vi "HUI.vi"() -> ()   [LabVIEW 2016]
uses:
  <vilib>/measure/NI_MABase.lvlib
panel:
  out "Point processed":u32
  in  "Quant":i32=100
  in  "stop":bool
  out "DAC FREQ/CH, Hz":dbl
  out "String":string
  in  "STOP_RUN":bool
  in  "FREQ":dbl(knob)=100.0 scale=0.0..100000.0
  in  "SIZE":dbl(knob)=1.0 scale=0.0..5.0
  # "CHANNEL A"
  # "CHANNEL B"
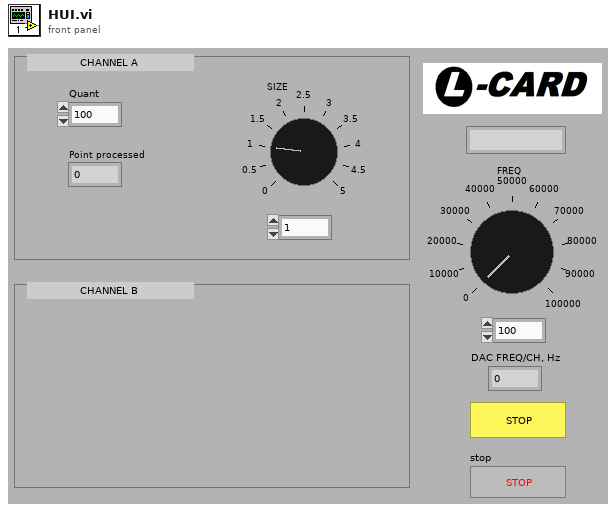
[diagram p1: front panel]
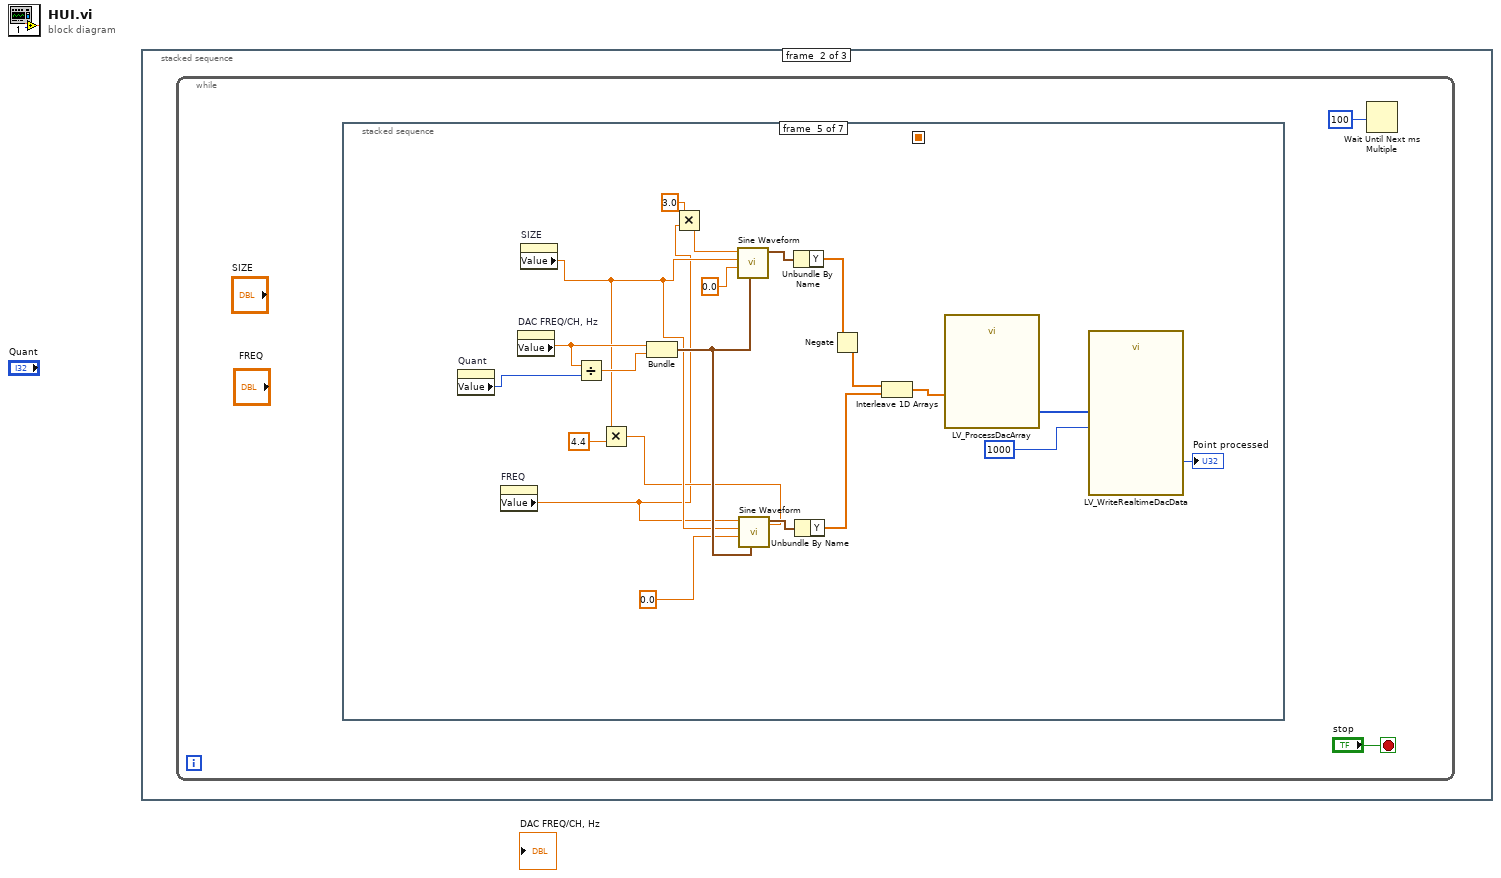
[diagram p0: block diagram]
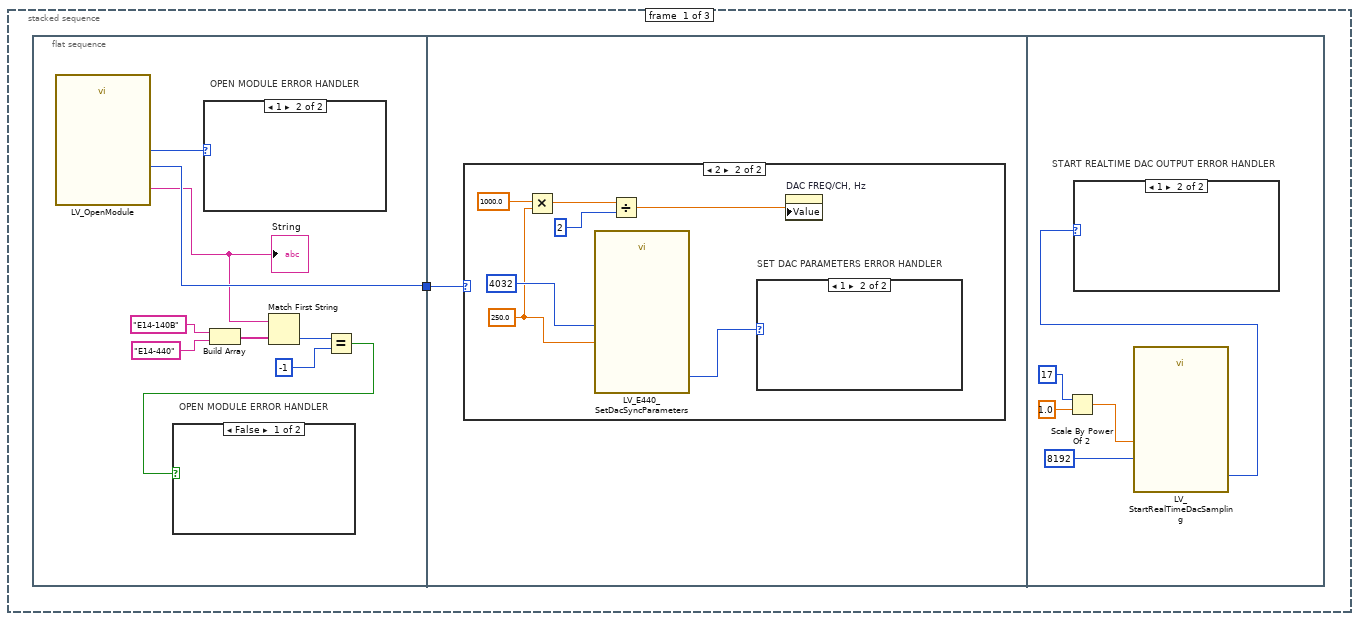
[diagram p2: hidden frame]
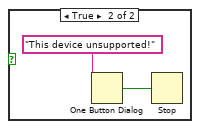
[diagram p3: hidden frame]
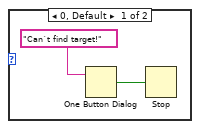
[diagram p4: hidden frame]
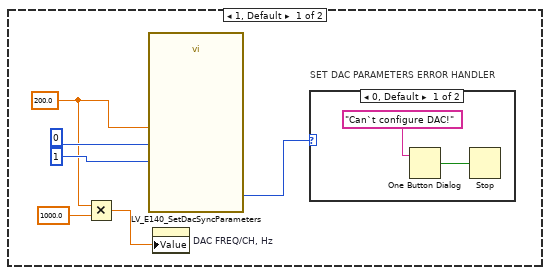
[diagram p5: hidden frame]
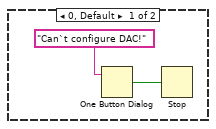
[diagram p7: hidden frame]
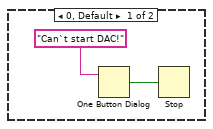
[diagram p8: hidden frame]
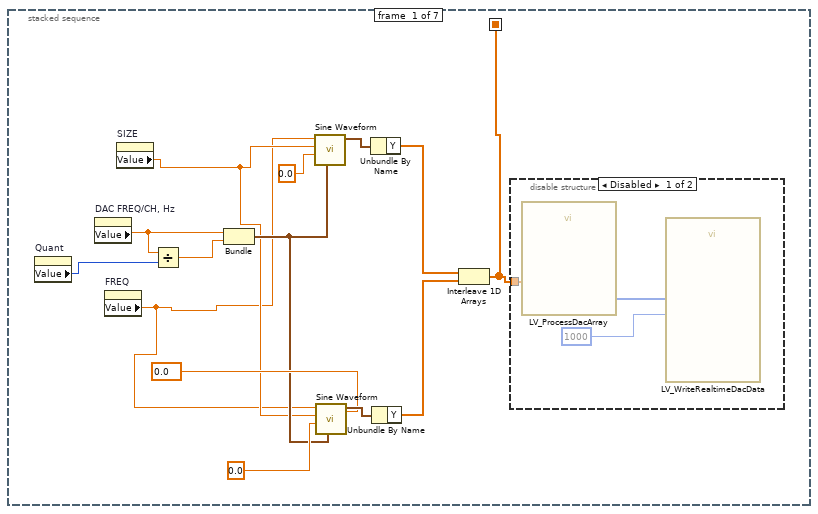
[diagram p9: hidden frame]
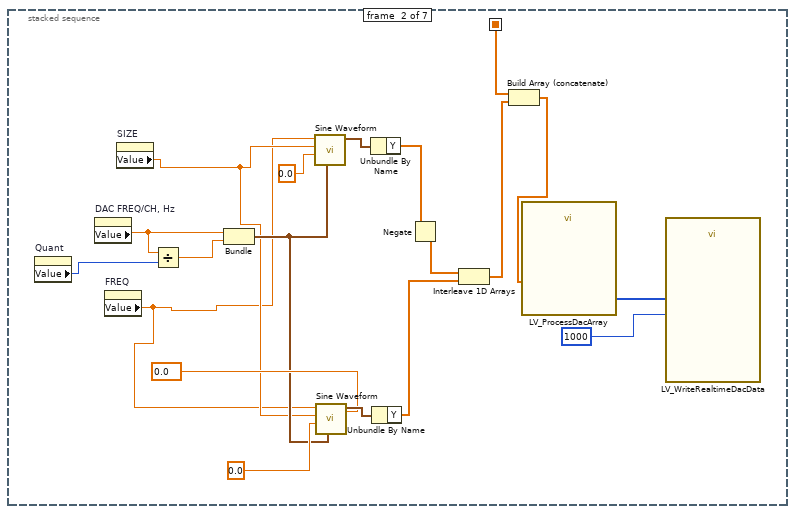
[diagram p11: hidden frame]
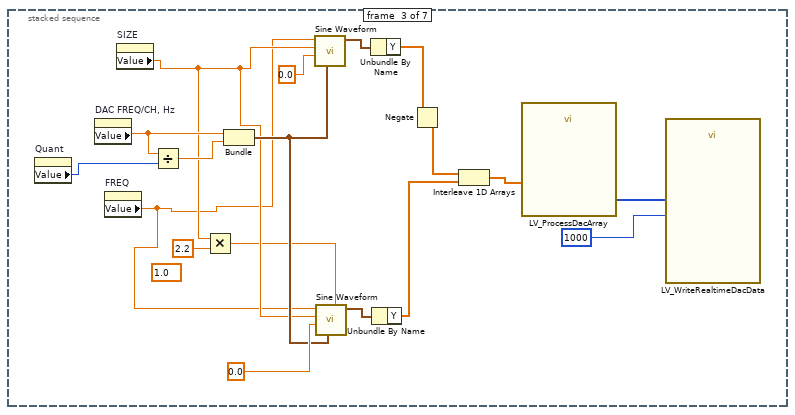
[diagram p12: hidden frame]
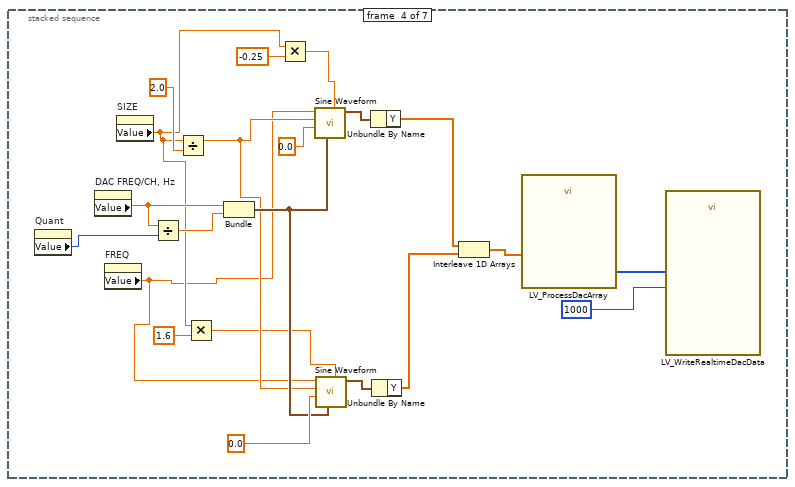
[diagram p13: hidden frame]
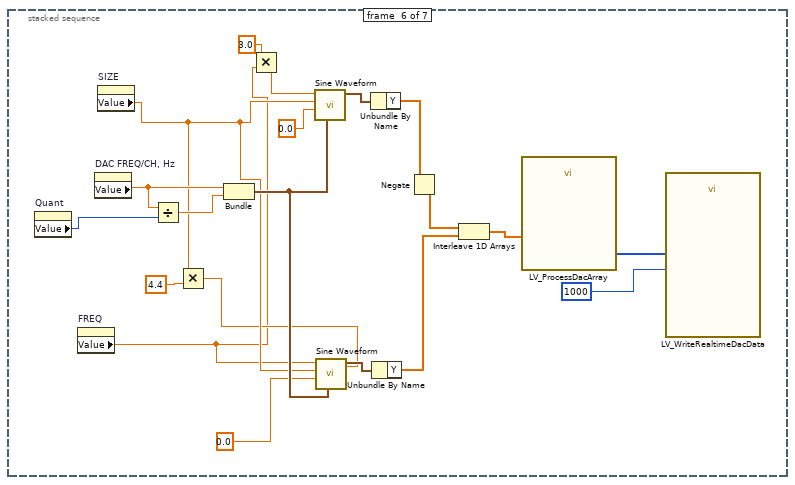
[diagram p14: hidden frame]
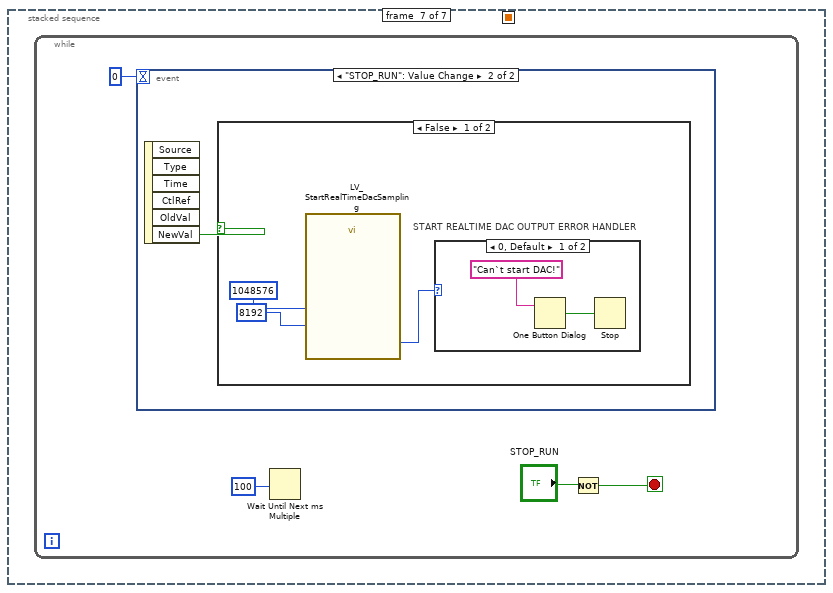
[diagram p15: hidden frame]
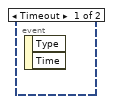
[diagram p16: hidden frame]
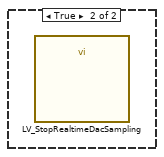
[diagram p18: hidden frame]
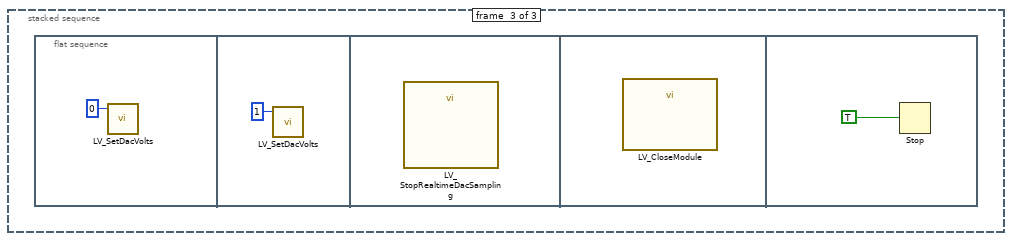
[diagram p19: hidden frame]
diagram:
  n1 = stacked-sequence {
    frame #0 {
      n2 = flat-sequence {
        tunnel: [w3] -> w1
        tunnel: w1 -> [w15]
        frame #0 {
          n3 = call <instrlib>:"LV_OpenModule.vi"() -> ("Module Name"=w2:string, "Module id"=w3:u8, "Error"=w4:u8)
          "String" <- w2
          n4 = case "OPEN MODULE ERROR HANDLER" shown="1" w4 {
            frame 0, Default {
              n5 = One Button Dialog(message="Can`t find target!") -> (true=w13:bool)  [unwired: 1 in]
              n6 = Stop(stop? (T)=w13) -> ()
            }
            frame 1 {
            }
          }
          n7 = Build Array("E14-140B", "E14-440") -> (w8:string[])
          n8 = Match First String(2:w8, 3:w2) -> (0:w7:i32)  [unwired: 1 out]
          n9 = Equal?(x=w7, y=-1) -> (x = y?=w5:bool)
          n10 = case "OPEN MODULE ERROR HANDLER" shown="False" w5 {
            frame False {
            }
            frame True {
              n11 = One Button Dialog(message="This device unsupported!") -> (true=w12:bool)  [unwired: 1 in]
              n12 = Stop(stop? (T)=w12) -> ()
            }
          }
        }
        frame #1 {
          n13 = case shown="2" w15 {
            frame 1, Default {
              w16 = 200.0
              n14 = Multiply(x=w16, y=1000.0) -> (x*y=w18:dbl)
              n15 = call <instrlib>:"LV_E140_SetDacSyncParameters.vi"("Zero on stop"=1, "Sync with ADC"=0, "Rate"=w16) -> ("Error"=w19:u32)  [unwired: 1 out]
              n16 = property on="DAC FREQ/CH, Hz" class="DigNum (strict)"("Value"=w18) -> ()  [unwired: 2 in, 2 out]
              n17 = case "SET DAC PARAMETERS ERROR HANDLER" shown="0, Default" w19 {
                frame 0, Default {
                  n18 = One Button Dialog(message="Can`t configure DAC!") -> (true=w22:bool)  [unwired: 1 in]
                  n19 = Stop(stop? (T)=w22) -> ()
                }
                frame 1 {
                }
              }
            }
            frame 2 {
              w25 = 250.0
              n20 = Multiply(x=1000.0, y=w25) -> (x*y=w26:dbl)
              n21 = call <instrlib>:"LV_E440_SetDacSyncParameters.vi"("Fifo length"=4032, "Rate"=w25) -> ("Error"=w27:u32)  [unwired: 1 out]
              n22 = Divide(x=w26, y=2) -> (x/y=w30:dbl)
              n23 = case "SET DAC PARAMETERS ERROR HANDLER" shown="1" w27 {
                frame 0, Default {
                  n24 = One Button Dialog(message="Can`t configure DAC!") -> (true=w31:bool)  [unwired: 1 in]
                  n25 = Stop(stop? (T)=w31) -> ()
                }
                frame 1 {
                }
              }
              n26 = property on="DAC FREQ/CH, Hz" class="DigNum (strict)"("Value"=w30) -> ()  [unwired: 2 in, 2 out]
            }
          }
        }
        frame #2 {
          n27 = Scale By Power Of 2(n=i16 17, x=1.0) -> (x*2^n=w33:dbl)
          n28 = call <instrlib>:"LV_StartRealTimeDacSampling.vi"("Packet size"=8192, "Buffer Size"=w33) -> ("Error"=w36:u8)
          n29 = case "START REALTIME DAC OUTPUT ERROR HANDLER" shown="1" w36 {
            frame 0, Default {
              n30 = One Button Dialog(message="Can`t start DAC!") -> (true=w38:bool)  [unwired: 1 in]
              n31 = Stop(stop? (T)=w38) -> ()
            }
            frame 1 {
            }
          }
        }
      }
    }
    frame #1 {
      n32 = while {
        stop <- "stop" stop-if-true
        n33 = stacked-sequence {
          seq-local: [w42 _ _ _ _ _ _] -> [_ w62 _ _ _ _ _]
          frame #0 {
            w52 = 0.0 items=["-5V"=-5.0, "-2V"=-2.0, "-1V"=-1.0, "0V"=0.0, "1V"=1.0, "2V"=2.0, "5V"=5.0] ("DC OFFSET")
            n34 = property on="Quant" class="DigNum (strict)"() -> ("Value"=w46:i32)  [unwired: 2 in, 2 out]
            n35 = property on="DAC FREQ/CH, Hz" class="DigNum (strict)"() -> ("Value"=w49:dbl)  [unwired: 2 in, 2 out]
            n36 = property on="FREQ" class="Knob (strict)"() -> ("Value"=w43:dbl)  [unwired: 2 in, 2 out]
            n37 = property on="SIZE" class="Knob (strict)"() -> ("Value"=w44:dbl)  [unwired: 2 in, 2 out]
            n38 = Divide(x=w49, y=w46) -> (x/y=w48:dbl)
            n39 = Bundle("Value"=w49, w48) -> (w45:cluster{"Value":dbl, dbl})  [unwired: 1 in]
            n40 = call <vilib>:"Sine Waveform.vi"("sampling info"=w45, "phase"=sgl 0.0, "amplitude"=w44, "frequency"=w43) -> ("signal out"=w55:waveform(dbl))  [unwired: 6 in, 1 out]
            n41 = call <vilib>:"Sine Waveform.vi"("offset"=w52, "sampling info"=w45, "phase"=0.0, "amplitude"=w44, "frequency"=w43) -> ("signal out"=w53:waveform(dbl))  [unwired: 5 in, 1 out]
            n42 = Unbundle By Name(w55) -> ("Y"=w51:dbl[])
            n43 = Unbundle By Name(w53) -> ("Y"=w50:dbl[])
            n44 = Interleave 1D Arrays(w51, w50) -> (w42:dbl[])
            n45 = disable-structure shown="Disabled" {
              disable-tunnel: w42 -> [w56 _]
              frame Disabled {
                n46 = call <instrlib>:"LV_ProcessDacArray.vi"("Input data"=w56) -> ("Output data"=w58:i16[])
                n47 = call <instrlib>:"LV_WriteRealtimeDacData.vi"("Timeout"=1000, "Data"=w58) -> ()  [unwired: 2 in, 3 out]
              }
              frame Enabled {
              }
            }
          }
          frame #1 {
            w74 = 0.0 items=["-5V"=-5.0, "-2V"=-2.0, "-1V"=-1.0, "0V"=0.0, "1V"=1.0, "2V"=2.0, "5V"=5.0] ("DC OFFSET")
            n48 = property on="Quant" class="DigNum (strict)"() -> ("Value"=w66:i32)  [unwired: 2 in, 2 out]
            n49 = property on="DAC FREQ/CH, Hz" class="DigNum (strict)"() -> ("Value"=w71:dbl)  [unwired: 2 in, 2 out]
            n50 = property on="FREQ" class="Knob (strict)"() -> ("Value"=w63:dbl)  [unwired: 2 in, 2 out]
            n51 = property on="SIZE" class="Knob (strict)"() -> ("Value"=w64:dbl)  [unwired: 2 in, 2 out]
            n52 = Divide(x=w71, y=w66) -> (x/y=w70:dbl)
            n53 = Bundle("Value"=w71, w70) -> (w65:cluster{"Value":dbl, dbl})  [unwired: 1 in]
            n54 = call <vilib>:"Sine Waveform.vi"("sampling info"=w65, "phase"=sgl 0.0, "amplitude"=w64, "frequency"=w63) -> ("signal out"=w77:waveform(dbl))  [unwired: 6 in, 1 out]
            n55 = call <vilib>:"Sine Waveform.vi"("offset"=w74, "sampling info"=w65, "phase"=0.0, "amplitude"=w64, "frequency"=w63) -> ("signal out"=w75:waveform(dbl))  [unwired: 5 in, 1 out]
            n56 = Unbundle By Name(w77) -> ("Y"=w73:dbl[])
            n57 = Unbundle By Name(w75) -> ("Y"=w72:dbl[])
            n58 = Negate(x=w73) -> (-x=w59:dbl[])
            n59 = Interleave 1D Arrays(w59, w72) -> (w61:dbl[])
            n60 = Build Array (concatenate)(w62, w61) -> (w60:dbl[])
            n61 = call <instrlib>:"LV_ProcessDacArray.vi"("Input data"=w60) -> ("Output data"=w69:i16[])
            n62 = call <instrlib>:"LV_WriteRealtimeDacData.vi"("Timeout"=1000, "Data"=w69) -> ()  [unwired: 2 in, 3 out]
          }
          frame #2 {
            (unwired) 1.0 items=["-5V"=-5.0, "-2V"=-2.0, "-1V"=-1.0, "0V"=0.0, "1V"=1.0, "2V"=2.0, "5V"=5.0] ("DC OFFSET")
            n63 = property on="Quant" class="DigNum (strict)"() -> ("Value"=w84:i32)  [unwired: 2 in, 2 out]
            n64 = property on="DAC FREQ/CH, Hz" class="DigNum (strict)"() -> ("Value"=w89:dbl)  [unwired: 2 in, 2 out]
            n65 = property on="FREQ" class="Knob (strict)"() -> ("Value"=w78:dbl)  [unwired: 2 in, 2 out]
            n66 = property on="SIZE" class="Knob (strict)"() -> ("Value"=w80:dbl)  [unwired: 2 in, 2 out]
            n67 = Divide(x=w89, y=w84) -> (x/y=w88:dbl)
            n68 = Multiply(x=w80, y=2.2) -> (x*y=w79:dbl)
            n69 = Bundle("Value"=w89, w88) -> (w83:cluster{"Value":dbl, dbl})  [unwired: 1 in]
            n70 = call <vilib>:"Sine Waveform.vi"("sampling info"=w83, "phase"=sgl 0.0, "amplitude"=w80, "frequency"=w78) -> ("signal out"=w95:waveform(dbl))  [unwired: 6 in, 1 out]
            n71 = call <vilib>:"Sine Waveform.vi"("offset"=w79, "sampling info"=w83, "phase"=0.0, "amplitude"=w80, "frequency"=w78) -> ("signal out"=w93:waveform(dbl))  [unwired: 5 in, 1 out]
            n72 = Unbundle By Name(w95) -> ("Y"=w92:dbl[])
            n73 = Unbundle By Name(w93) -> ("Y"=w91:dbl[])
            n74 = Negate(x=w92) -> (-x=w82:dbl[])
            n75 = Interleave 1D Arrays(w82, w91) -> (w90:dbl[])
            n76 = call <instrlib>:"LV_ProcessDacArray.vi"("Input data"=w90) -> ("Output data"=w87:i16[])
            n77 = call <instrlib>:"LV_WriteRealtimeDacData.vi"("Timeout"=1000, "Data"=w87) -> ()  [unwired: 2 in, 3 out]
          }
          frame #3 {
            n78 = property on="Quant" class="DigNum (strict)"() -> ("Value"=w105:i32)  [unwired: 2 in, 2 out]
            n79 = property on="DAC FREQ/CH, Hz" class="DigNum (strict)"() -> ("Value"=w110:dbl)  [unwired: 2 in, 2 out]
            n80 = property on="FREQ" class="Knob (strict)"() -> ("Value"=w96:dbl)  [unwired: 2 in, 2 out]
            n81 = property on="SIZE" class="Knob (strict)"() -> ("Value"=w98:dbl)  [unwired: 2 in, 2 out]
            n82 = Divide(x=w110, y=w105) -> (x/y=w109:dbl)
            n83 = Divide(x=w98, y=2.0) -> (x/y=w103:dbl)
            n84 = Multiply(x=w98, y=1.6) -> (x*y=w100:dbl)
            n85 = Bundle("Value"=w110, w109) -> (w104:cluster{"Value":dbl, dbl})  [unwired: 1 in]
            n86 = Multiply(x=w98, y=-0.25) -> (x*y=w97:dbl)
            n87 = call <vilib>:"Sine Waveform.vi"("offset"=w97, "sampling info"=w104, "phase"=sgl 0.0, "amplitude"=w103, "frequency"=w96) -> ("signal out"=w116:waveform(dbl))  [unwired: 5 in, 1 out]
            n88 = call <vilib>:"Sine Waveform.vi"("offset"=w100, "sampling info"=w104, "phase"=0.0, "amplitude"=w103, "frequency"=w96) -> ("signal out"=w114:waveform(dbl))  [unwired: 5 in, 1 out]
            n89 = Unbundle By Name(w116) -> ("Y"=w113:dbl[])
            n90 = Unbundle By Name(w114) -> ("Y"=w112:dbl[])
            n91 = Interleave 1D Arrays(w113, w112) -> (w111:dbl[])
            n92 = call <instrlib>:"LV_ProcessDacArray.vi"("Input data"=w111) -> ("Output data"=w108:i16[])
            n93 = call <instrlib>:"LV_WriteRealtimeDacData.vi"("Timeout"=1000, "Data"=w108) -> ()  [unwired: 2 in, 3 out]
          }
          frame #4 {
            n94 = property on="Quant" class="DigNum (strict)"() -> ("Value"=w127:i32)  [unwired: 2 in, 2 out]
            n95 = property on="FREQ" class="Knob (strict)"() -> ("Value"=w119:dbl)  [unwired: 2 in, 2 out]
            n96 = property on="DAC FREQ/CH, Hz" class="DigNum (strict)"() -> ("Value"=w131:dbl)  [unwired: 2 in, 2 out]
            n97 = property on="SIZE" class="Knob (strict)"() -> ("Value"=w123:dbl)  [unwired: 2 in, 2 out]
            n98 = Divide(x=w131, y=w127) -> (x/y=w130:dbl)
            n99 = Multiply(x=w123, y=4.4) -> (x*y=w122:dbl)
            n100 = Bundle("Value"=w131, w130) -> (w126:cluster{"Value":dbl, dbl})  [unwired: 1 in]
            n101 = Multiply(x=3.0 ("frequency"), y=w119) -> (x*y=w120:dbl)
            n102 = call <vilib>:"Sine Waveform.vi"("sampling info"=w126, "phase"=sgl 0.0, "amplitude"=w123, "frequency"=w120) -> ("signal out"=w137:waveform(dbl))  [unwired: 6 in, 1 out]
            n103 = call <vilib>:"Sine Waveform.vi"("offset"=w122, "sampling info"=w126, "phase"=0.0, "amplitude"=w123, "frequency"=w119) -> ("signal out"=w135:waveform(dbl))  [unwired: 5 in, 1 out]
            n104 = Unbundle By Name(w137) -> ("Y"=w134:dbl[])
            n105 = Unbundle By Name(w135) -> ("Y"=w133:dbl[])
            n106 = Negate(x=w134) -> (-x=w118:dbl[])
            n107 = Interleave 1D Arrays(w118, w133) -> (w132:dbl[])
            n108 = call <instrlib>:"LV_ProcessDacArray.vi"("Input data"=w132) -> ("Output data"=w129:i16[])
            n109 = call <instrlib>:"LV_WriteRealtimeDacData.vi"("Timeout"=1000, "Data"=w129) -> ("Point processed"=→"Point processed":u32)  [unwired: 2 in, 2 out]
          }
          frame #5 {
            n110 = property on="Quant" class="DigNum (strict)"() -> ("Value"=w147:i32)  [unwired: 2 in, 2 out]
            n111 = property on="FREQ" class="Knob (strict)"() -> ("Value"=w139:dbl)  [unwired: 2 in, 2 out]
            n112 = property on="DAC FREQ/CH, Hz" class="DigNum (strict)"() -> ("Value"=w151:dbl)  [unwired: 2 in, 2 out]
            n113 = property on="SIZE" class="Knob (strict)"() -> ("Value"=w143:dbl)  [unwired: 2 in, 2 out]
            n114 = Divide(x=w151, y=w147) -> (x/y=w150:dbl)
            n115 = Multiply(x=w143, y=4.4) -> (x*y=w142:dbl)
            n116 = Bundle("Value"=w151, w150) -> (w146:cluster{"Value":dbl, dbl})  [unwired: 1 in]
            n117 = Multiply(x=3.0 ("frequency"), y=w139) -> (x*y=w140:dbl)
            n118 = call <vilib>:"Sine Waveform.vi"("sampling info"=w146, "phase"=sgl 0.0, "amplitude"=w143, "frequency"=w140) -> ("signal out"=w157:waveform(dbl))  [unwired: 6 in, 1 out]
            n119 = call <vilib>:"Sine Waveform.vi"("offset"=w142, "sampling info"=w146, "phase"=0.0, "amplitude"=w143, "frequency"=w139) -> ("signal out"=w155:waveform(dbl))  [unwired: 5 in, 1 out]
            n120 = Unbundle By Name(w157) -> ("Y"=w154:dbl[])
            n121 = Unbundle By Name(w155) -> ("Y"=w153:dbl[])
            n122 = Negate(x=w154) -> (-x=w138:dbl[])
            n123 = Interleave 1D Arrays(w138, w153) -> (w152:dbl[])
            n124 = call <instrlib>:"LV_ProcessDacArray.vi"("Input data"=w152) -> ("Output data"=w149:i16[])
            n125 = call <instrlib>:"LV_WriteRealtimeDacData.vi"("Timeout"=1000, "Data"=w149) -> ()  [unwired: 2 in, 3 out]
          }
          frame #6 {
            n126 = while {
              stop <- w158 stop-if-true
              n127 = event shown="[1] \"STOP_RUN\": Value Change" {
                selector: _ -> [_ _]
                dyn-events: _ -> [_ _]
                timeout: 0 -> [_ _]
                event Timeout {
                  n128 = event-data() -> ()  [unwired: 1 in, 2 out]
                }
                event "STOP_RUN": Value Change {
                  n129 = event-data() -> ("NewVal"=w162:bool)  [unwired: 1 in, 5 out]
                  n130 = case shown="False" w162 {
                    frame False {
                      n131 = call <instrlib>:"LV_StartRealTimeDacSampling.vi"("Packet size"=8192, "Buffer Size"=1048576) -> ("Error"=w163:u8)
                      n132 = case "START REALTIME DAC OUTPUT ERROR HANDLER" shown="0, Default" w163 {
                        frame 0, Default {
                          n133 = One Button Dialog(message="Can`t start DAC!") -> (true=w166:bool)  [unwired: 1 in]
                          n134 = Stop(stop? (T)=w166) -> ()
                        }
                        frame 1 {
                        }
                      }
                    }
                    frame True {
                      n135 = call <instrlib>:"LV_StopRealtimeDacSampling.vi"() -> ()  [unwired: 1 in]
                    }
                  }
                }
              }
              n136 = Wait Until Next ms Multiple(millisecond multiple=100) -> ()  [unwired: 1 out]
              n137 = Not(x="STOP_RUN") -> (.not. x?=w158:bool)
            }
          }
        }
        n138 = Wait Until Next ms Multiple(millisecond multiple=100) -> ()  [unwired: 1 out]
      }
    }
    frame #2 {
      n139 = flat-sequence {
        frame #0 {
          n140 = call <instrlib>:"LV_SetDacVolts.vi"("Channel Num"=u32 0) -> ()  [unwired: 2 in]
        }
        frame #1 {
          n141 = call <instrlib>:"LV_SetDacVolts.vi"("Channel Num"=u32 1) -> ()  [unwired: 2 in]
        }
        frame #2 {
          n142 = call <instrlib>:"LV_StopRealtimeDacSampling.vi"() -> ()  [unwired: 1 in]
        }
        frame #3 {
          n143 = call <instrlib>:"LV_CloseModule.vi"() -> ()  [unwired: 1 in]
        }
        frame #4 {
          n144 = Stop(stop? (T)=TRUE) -> ()
        }
      }
    }
  }
